vi "Load Demos.vi"(7 "Top Level Folder Order":string[](array[string]), 8 "error in":errorcluster, 10 "Tree":refnum<vi>, 11 "Ignored Demos":string[](array[string])) -> (0 "error out":errorcluster, 3 "Demos":T1)   [LabVIEW 2020]
uses:
  Demo_class/Demo.lvclass
  Interactive_class/Interactive.lvclass
  C:/dev/github/labview-demo-station/LabVIEW Demo Station/support/Demo_class/Demo.lvclass
  Passive_class/Passive.lvclass
  Demo_class/Demo.lvclass/Demo.ctl
  Tree Tag to Demo--map.ctl
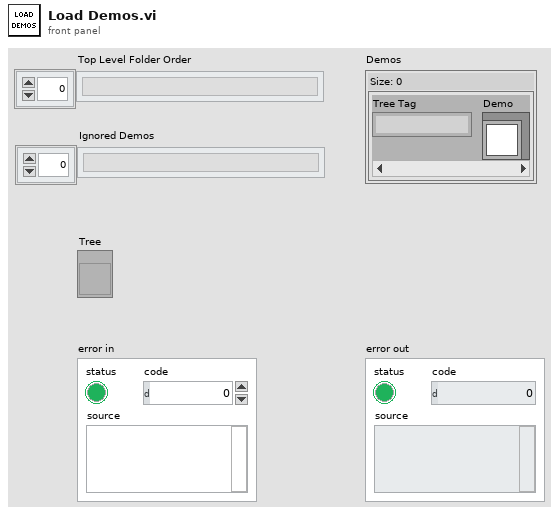
[diagram p1: front panel]
types:
  T1 = typedef "Tree Tag to Demo--map.ctl" = map{string, refnum<class "Demo.lvclass">}
  T2 = typedef "imagedata.ctl" = cluster{"image type":i32, "image depth":i32, "image":u8[], "mask":u8[], "colors":u32[], "Rectangle":cluster{"left":i16, "top":i16, "right":i16, "bottom":i16}}
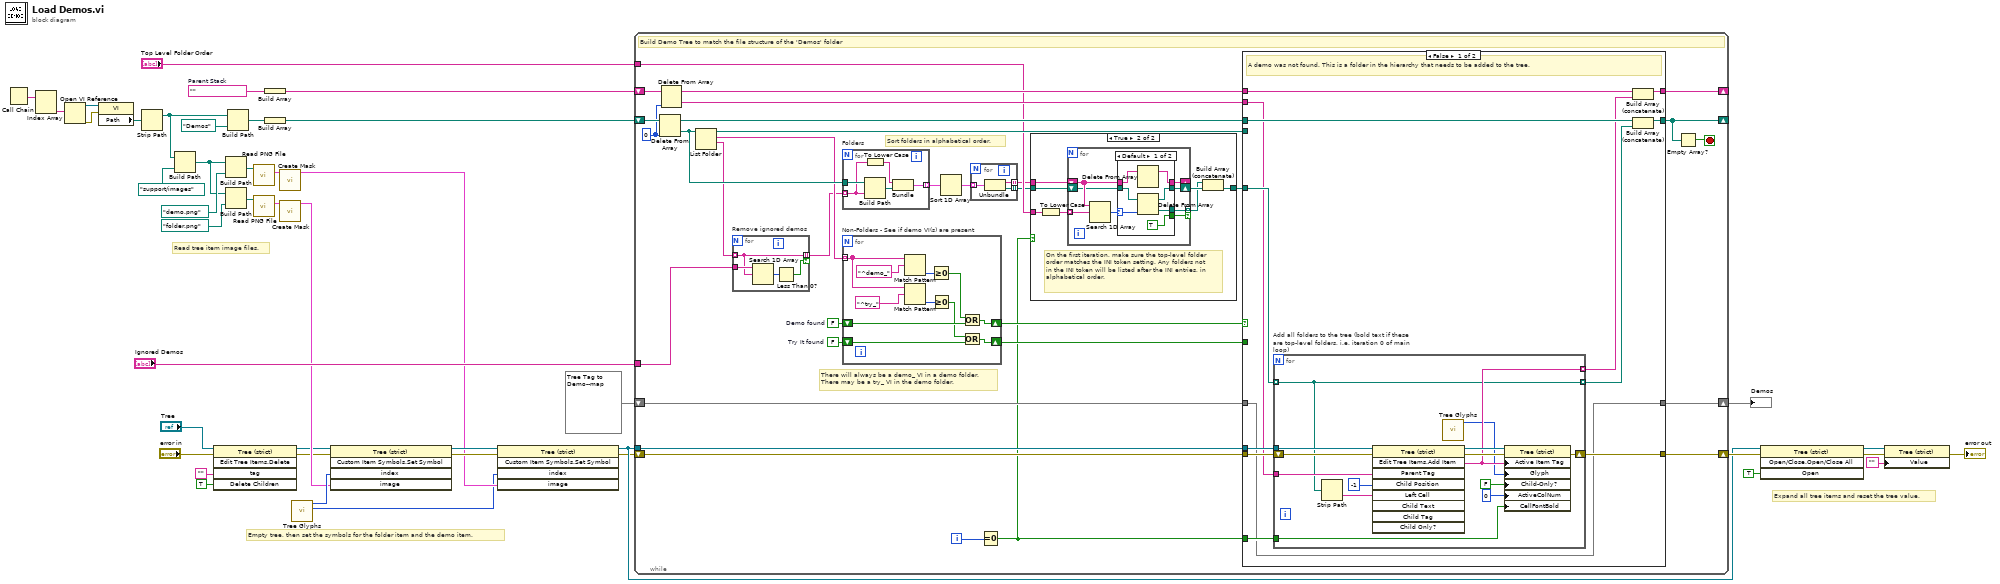
[diagram p0: block diagram]
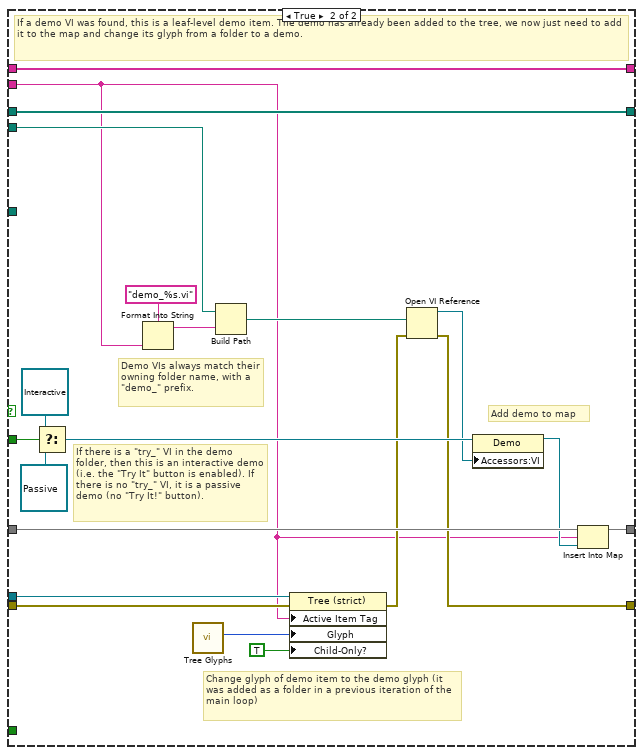
[diagram p4: hidden frame]
diagram:
  w39 = ""  # Parent Stack
  # "Expand all tree items and reset the tree value."
  # "Empty tree, then set the symbols for the folder item and the demo item."
  # "Read tree item image files."
  n1 = Call Chain() -> (call chain=w6:string[])
  n2 = Index Array(array=w6) -> (element #2=w5:string)  [unwired: 2 in, 1 out]
  n3 = Open VI Reference(vi path=w5) -> (vi reference=w4:refnum<vi>, error out=w2:errorcluster)  [unwired: 5 in]
  n4 = property class="VI"(reference=w4, error in=w2) -> ("Path"=w3:path)  [unwired: 2 out]
  n5 = Strip Path(path=w3) -> (stripped path=w1:path)  [unwired: 1 out]
  n6 = Build Path(base path=w1, name or relative path=path "support/images") -> (appended path=w19:path)
  n7 = invoke class="Tree (strict)" method="Edit Tree Items.Delete"(reference="Tree", error in="error in", "tag"="", "Delete Children"=TRUE) -> (reference out=w9:refnum<vi>, error out=w11:errorcluster)  [unwired: 1 in, 3 out]
  n8 = Build Path(base path=w19, name or relative path=path "demo.png") -> (appended path=w21:path)
  n9 = Build Path(base path=w19, name or relative path=path "folder.png") -> (appended path=w27:path)
  n10 = Build Path(base path=w1, name or relative path=path "Demos") -> (appended path=w38:path)
  n11 = call <vilib>:"Read PNG File.vi"("path to PNG file"=w21) -> ("image data"=w18:T2)  [unwired: 8 in, 2 out]
  n12 = call <vilib>:"Read PNG File.vi"("path to PNG file"=w27) -> ("image data"=w16:T2)  [unwired: 8 in, 2 out]
  n13 = Build Array(w39) -> (w37:string[])
  n14 = Build Array(w38) -> (w35:path[])
  n15 = call <vilib>:"Create Mask.vi"("image data"=w18) -> ("image data"=w17:T2)  [unwired: 10 in]
  n16 = call <vilib>:"Create Mask.vi"("image data"=w16) -> ("image data"=w15:T2)  [unwired: 10 in]
  n17 = call "Tree Glyphs.vi"() -> ("Demo Glyph Index"=w13:i32, "Folder Glyph Index"=w26:i32)  [unwired: 10 in]
  n18 = invoke class="Tree (strict)" method="Custom Item Symbols.Set Symbol"(reference=w9, error in=w11, "index"=w26, "image"=w15) -> (reference out=w25:refnum<vi>, error out=w24:errorcluster)  [unwired: 1 in, 3 out]
  n19 = invoke class="Tree (strict)" method="Custom Item Symbols.Set Symbol"(reference=w25, error in=w24, "index"=w13, "image"=w17) -> (reference out=w23:refnum<vi>, error out=w22:errorcluster)  [unwired: 1 in, 3 out]
  n20 = while {
    shift-right: [w64] -> w43
    shift-left: w22 -> [w66]
    tunnel: "Ignored Demos" -> [w51]
    shift-right: [w68] -> w40
    shift-left: T1 {} ("Map") -> [w67]
    shift-right: [w63] -> _
    shift-left: w37 -> [w62]
    shift-right: [w60] -> _
    shift-left: w35 -> [w75]
    tunnel: w23 -> [w65]
    tunnel: "Top Level Folder Order" -> [w47]
    i -> [w50]
    stop <- w59 stop-if-true
    w55 = 0 ("index")
    w71 = FALSE  # Try It found
    w72 = FALSE  # Demo found
    # "There will always be a demo_ VI in a demo folder.\nThere may be a try_ VI in the demo folder."
    # "Sort folders in alphabetical order."
    # "Build Demo Tree to match the file structure of the 'Demos' folder"
    n21 = Delete From Array(array=w75, index=w55) -> (deleted portion=w74:path, array with subset deleted=w61:path[])  [unwired: 1 in]
    n22 = Delete From Array(array=w62, index=w55) -> (deleted portion=w57:string, array with subset deleted=w58:string[])  [unwired: 1 in]
    n23 = List Folder(path=w74) -> (path out=w54:path, filenames=w73:string[], folder names=w53:string[])  [unwired: 3 in, 1 out]
    n24 = for "Remove ignored demos" {
      tunnel: [w106] -> w52 mode=indexing if=w104
      tunnel: w53 -> [w106] mode=indexing
      tunnel: w51 -> [w107]
      n25 = Search 1D Array(1D array=w107, element=w106) -> (index of element=w105:i32)  [unwired: 1 in]
      n26 = Less Than 0?(x=w105) -> (x < 0?=w104:bool)
    }
    n27 = for "Folders" {
      tunnel: w52 -> [w168] mode=indexing
      tunnel: w74 -> [w171]
      tunnel: [w169] -> w56 mode=indexing
      n28 = To Lower Case(string=w168) -> (all lower case string=w167:string)
      n29 = Build Path(base path=w171, name or relative path=w168) -> (appended path=w170:path)
      n30 = Bundle(w167, "appended path"=w170) -> (w169:cluster{string, "appended path":path})  [unwired: 1 in]
    }
    n31 = for "Non-Folders - See if demo VI(s) are present" {
      tunnel: w73 -> [w162] mode=indexing
      shift-right: [w165] -> w70
      shift-left: w72 -> [w166]
      shift-right: [w163] -> w69
      shift-left: w71 -> [w164]
      n32 = Match Pattern(string=w162, regular expression="^demo_") -> (offset past match=w159:i32)  [unwired: 1 in, 3 out]
      n33 = Match Pattern(string=w162, regular expression="^try_") -> (offset past match=w157:i32)  [unwired: 1 in, 3 out]
      n34 = Greater Or Equal To 0?(x=w159) -> (x >= 0?=w158:bool)
      n35 = Greater Or Equal To 0?(x=w157) -> (x >= 0?=w156:bool)
      n36 = Or(x=w158, y=w166) -> (x .or. y?=w165:bool)
      n37 = Or(x=w156, y=w164) -> (x .or. y?=w163:bool)
    }
    n38 = Sort 1D Array(array=w56) -> (sorted array=w46:cluster{string, "appended path":path}[])
    n39 = for {
      tunnel: w46 -> [w78] mode=indexing
      tunnel: [w77] -> w44 mode=indexing
      tunnel: [w76] -> w45 mode=indexing
      n40 = Unbundle(w78) -> (w76:string, "appended path"=w77:path)
    }
    n41 = Equal To 0?(x=w50) -> (x = 0?=w49:bool)
    n42 = case shown="True" w49 {
      tunnel: [w79 w81] -> w48
      tunnel: w47 -> [_ w86]
      tunnel: w45 -> [_ w84]
      tunnel: w44 -> [w79 w83]
      frame False {
        # "All non-top-level folders are sorted in alphabetical order."
      }
      frame True {
        # "On the first iteration, make sure the top-level folder order matches the INI token setting. Any folders not in the INI token will be listed after the INI entries, in alphabetical order."
        n43 = To Lower Case(string=w86) -> (all lower case string=w85:string[])
        n44 = for {
          tunnel: w85 -> [w94] mode=indexing
          shift-right: [w92] -> _
          shift-left: w84 -> [w91]
          shift-right: [w90] -> w82
          shift-left: w83 -> [w89]
          tunnel: [w88] -> w80 mode=indexing if=w87
          n45 = Search 1D Array(1D array=w91, element=w94) -> (index of element=w93:i32)  [unwired: 1 in]
          n46 = case shown="Default" w93 {
            selector: w93 -> [w98 _]
            tunnel: [w100 w103] -> w92
            tunnel: w91 -> [w101 w103]
            tunnel: [w97 w102] -> w90
            tunnel: w89 -> [w99 w102]
            tunnel: [w96 _] -> w88
            tunnel: [TRUE _] -> w87
            frame Default {
              n47 = Delete From Array(array=w101) -> (array with subset deleted=w100:string[])  [unwired: 2 in, 1 out]
              n48 = Delete From Array(array=w99, index=w98) -> (deleted portion=w96:path, array with subset deleted=w97:path[])  [unwired: 1 in]
            }
            frame -1 {
            }
          }
        }
        n49 = Build Array (concatenate)(w80, w82) -> (w81:path[])
      }
    }
    n50 = case shown="False" w70 {
      tunnel: w69 -> [_ w155]
      tunnel: [w108 w151] -> w68
      tunnel: w67 -> [w108 w152]
      tunnel: w66 -> [w115 w140]
      tunnel: w65 -> [w114 w138]
      tunnel: [w113 w145] -> w64
      tunnel: [w117 w149] -> w63
      tunnel: w58 -> [w118 w149]
      tunnel: w61 -> [w120 w148]
      tunnel: [w119 w148] -> w60
      tunnel: w57 -> [w110 w137]
      tunnel: w48 -> [w116 _]
      tunnel: w54 -> [_ w143]
      tunnel: w49 -> [w109 _]
      frame False {
        # "A demo was not found. This is a folder in the hierarchy that needs to be added to the tree."
        n51 = for "Add all folders to the tree (bold text if these are top-level folders, i.e. iteration 0 of main loop)" {
          tunnel: w116 -> [w122] mode=indexing
          shift-right: [w128] -> w113
          shift-left: w115 -> [w134]
          tunnel: w114 -> [w133]
          tunnel: [w126] -> w112 mode=indexing
          tunnel: [w122] -> w111 mode=indexing
          tunnel: w110 -> [w131]
          tunnel: w109 -> [w123]
          n52 = Strip Path(path=w122) -> (name=w130:string)  [unwired: 1 out]
          n53 = invoke class="Tree (strict)" method="Edit Tree Items.Add Item"(reference=w133, error in=w134, "Parent Tag"=w131, "Child Position"=-1, "Left Cell"=w130) -> (reference out=w127:refnum<vi>, error out=w132:errorcluster, "Edit Tree Items:Add Item"=w126:string)  [unwired: 4 in, 6 out]
          n54 = call "Tree Glyphs.vi"() -> ("Folder Glyph Index"=w121:i32)  [unwired: 10 in, 1 out]
          n55 = property class="Tree (strict)"(reference=w127, error in=w132, "Active Item Tag"=w126, "Glyph"=w121, "Child-Only?"=FALSE ("Active Item:Child-Only?"), "ActiveColNum"=0 ("Active Cell:Active Column Number"), "CellFontBold"=w123) -> (error out=w128:errorcluster)  [unwired: 1 out]
        }
        n56 = Build Array (concatenate)(w118, w112) -> (w117:string[])
        n57 = Build Array (concatenate)(w120, w111) -> (w119:path[])
      }
      frame True {
        # "If there is a \"try_\" VI in the demo folder, then this is an interactive demo (i.e. the \"Try It\" button is enabled). If there is no \"try_\" VI, it is a passive demo (no \"Try It!\" button)."
        # "Demo VIs always match their owning folder name, with a \"demo_\" prefix."
        # "Add demo to map"
        # "Change glyph of demo item to the demo glyph (it was added as a folder in a previous iteration of the main loop)"
        # "If a demo VI was found, this is a leaf-level demo item. The demo has already been added to the tree, we now just need to add it to the map and change its glyph from a folder to a demo."
        n58 = Select(t=refnum<class "Interactive.lvclass"> refnum ("Interactive"), s=w155, f=refnum<class "Passive.lvclass"> refnum ("Passive")) -> (s? t:f=w150:refnum<class "Demo.lvclass">)
        n59 = Format Into String(format string="demo_%s.vi", w137) -> (resulting string=w142:string)  [unwired: 2 in, 1 out]
        n60 = call "Tree Glyphs.vi"() -> ("Demo Glyph Index"=w135:i32)  [unwired: 10 in, 1 out]
        n61 = Build Path(base path=w143, name or relative path=w142) -> (appended path=w144:path)
        n62 = property class="Tree (strict)"(reference=w138, error in=w140, "Active Item Tag"=w137, "Glyph"=w135, "Child-Only?"=TRUE ("Active Item:Child-Only?")) -> (error out=w139:errorcluster)  [unwired: 1 out]
        n63 = Open VI Reference(vi path=w144, error in (no error)=w139) -> (vi reference=w146:refnum<vi>, error out=w145:errorcluster)  [unwired: 4 in]
        n64 = property class="Demo"(reference=w150, "Accessors:VI"=w146) -> (reference out=w147:refnum<class "Demo.lvclass">)  [unwired: 1 in, 1 out]
        n65 = Insert Into Map(map in=w152, key=w137, value=w147) -> (map out=w151:T1)  [unwired: 2 out]
      }
    }
    n66 = Empty Array?(array=w60) -> (empty?=w59:bool)
  }
  "Demos" <- w40
  n67 = invoke class="Tree (strict)" method="Open/Close.Open/Close All"(reference=w23, error in=w43, "Open"=TRUE ("Open?")) -> (reference out=w31:refnum<vi>, error out=w34:errorcluster)  [unwired: 1 in, 2 out]
  n68 = property class="Tree (strict)"(reference=w31, error in=w34, "Value"="") -> (error out=→"error out":errorcluster)  [unwired: 1 out]
